vi "TDT-Set Run Mode.vi"(0 "Data":T3={"TTankX"=refnum, "TDevAccX"=refnum, "LastTime"=0.0, "error"={"status"=FALSE, "code"=0, "source"=""}, "Block Name"="", "Circuit Tag"="", "Tank Name"="", "NumTicks"=0, "LastTick"=0.0, "Idle?"=FALSE, "Wait (ms)"=1000, "LastArtf"=0.0, "LastTosc"=0.0}, 1 "Close Tank?":bool=TRUE, 7 "Trigger Source":T2, 11 "error in (no error)":errorcluster, 12 "OpenEx mode":T1) -> (4 "Data out":T3={"TTankX"=refnum, "TDevAccX"=refnum, "LastTime"=0.0, "error"={"status"=FALSE, "code"=0, "source"=""}, "Block Name"="", "Circuit Tag"="", "Tank Name"="", "NumTicks"=0, "LastTick"=0.0, "Idle?"=FALSE, "Wait (ms)"=1000, "LastArtf"=0.0, "LastTosc"=0.0}, 15 "error out":errorcluster)   [LabVIEW 2015]
uses:
  TDT Interface Data.ctl
  TDT-Trigger Source Enum.ctl
  TDT-Sys Mode Enum.ctl
  TDT-Set Target Val (DBL).vi
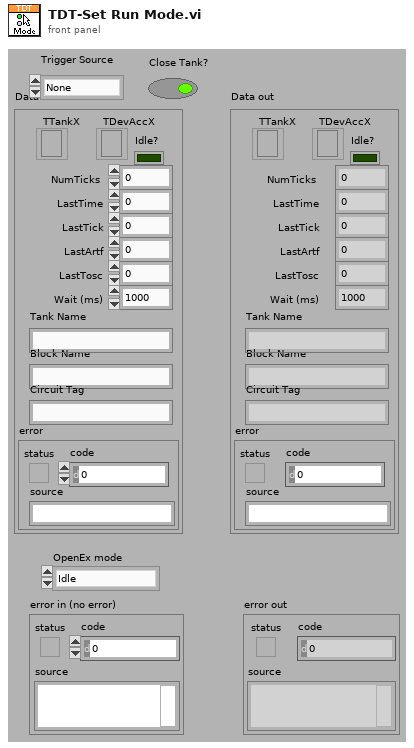
[diagram p1: front panel]
types:
  T1 = typedef "TDT-Sys Mode Enum.ctl" = enum16{"Idle", "Standby", "Preview", "Record"}
  T2 = typedef "TDT-Trigger Source Enum.ctl" = enum16{"None", "Impale", "Tosca", "PTB"}
  T3 = typedef "TDT Interface Data.ctl" = cluster{"TTankX":refnum<k7>, "TDevAccX":refnum<k7>, "LastTime":dbl, "error":errorcluster, "Block Name":string, "Circuit Tag":string, "Tank Name":string, "NumTicks":i32, "LastTick":dbl, "Idle?":bool, "Wait (ms)":u32, "LastArtf":dbl, "LastTosc":dbl}
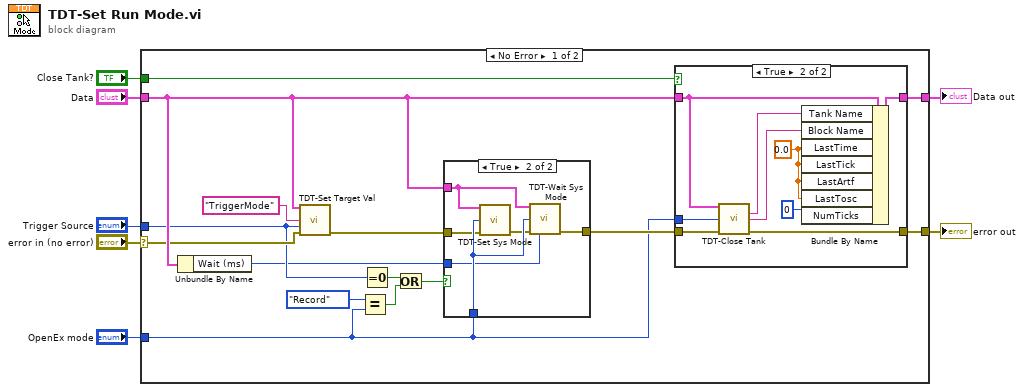
[diagram p0: block diagram]
diagram:
  n1 = case shown="No Error" "error in (no error)" {
    selector: "error in (no error)" -> [w16 w41]
    tunnel: "Data" -> [w18 w42]
    tunnel: "Trigger Source" -> [w15 _]
    tunnel: [w21 w42] -> w4
    tunnel: [w22 w41] -> w3
    tunnel: "OpenEx mode" -> [w13 _]
    tunnel: "Close Tank?" -> [w8 _]
    frame No Error {
      n2 = Unbundle By Name(w18) -> ("Wait (ms)"=w9:u32)
      n3 = call-poly "TDT-Set Target Val.vi"("Data"=w18, "Target"="TriggerMode", "Val"=w15, "error in (no error)"=w16) -> ("error out"=w19:errorcluster)  [unwired: 11 in]
      n4 = Equal?(x=TDT-Sys_Mode_Enum."Record", y=w13) -> (x = y?=w14:bool)
      n5 = Equal To 0?(x=w15) -> (x = 0?=w10:bool)
      n6 = Or(x=w10, y=w14) -> (x .or. y?=w11:bool)
      n7 = case shown="True" w11 {
        tunnel: w13 -> [_ w40]
        tunnel: [w34 w38] -> w20
        tunnel: w19 -> [w34 w37]
        tunnel: w18 -> [_ w36]
        tunnel: w9 -> [_ w35]
        frame False {
        }
        frame True {
          n8 = call "TDT-Set Sys Mode.vi"("Data"=w36, "NewMode"=w40, "error in (no error)"=w37) -> ("error out"=w39:errorcluster)  [unwired: 12 in]
          n9 = call "TDT-Wait Sys Mode.vi"("Data"=w36, "NewMode"=w40, "error in (no error)"=w39, "milliseconds to wait"=w35) -> ("error out"=w38:errorcluster)  [unwired: 11 in]
        }
      }
      n10 = case shown="True" w8 {
        tunnel: [w23 w32] -> w22
        tunnel: [w24 w31] -> w21
        tunnel: w20 -> [w23 w28]
        tunnel: w18 -> [w24 w27]
        tunnel: w13 -> [_ w26]
        frame False {
        }
        frame True {
          w25 = 0.0 ("LastTime")
          n11 = call "TDT-Close Tank.vi"("Data"=w27, "Mode"=w26, "error in (no error)"=w28) -> ("TankName"=w30:string, "Block Name"=w33:string, "error out"=w32:errorcluster)  [unwired: 10 in]
          n12 = Bundle By Name(cluster=w27, "Tank Name"=w30, "Block Name"=w33, "LastTime"=w25, "LastTick"=w25, "LastArtf"=w25, "LastTosc"=w25, "NumTicks"=0) -> (w31:T3)
        }
      }
    }
    frame Error {
    }
  }
  "error out" <- w3
  "Data out" <- w4
